vi "New plot.vi"() -> (0 "Boolean":bool)   [LabVIEW 2021]
uses:
  <vilib>/Utility/file.llb/Read Delimited Spreadsheet (string).vi
panel:
  out "filename":string
  out "VI Clone Name":string
  in  "file path (dialog if empty)":path
  out "XY Graph":cluster{dbl[], dbl[]}(graph)
  in  "stop":bool
  in  "Listbox":i32(listbox)
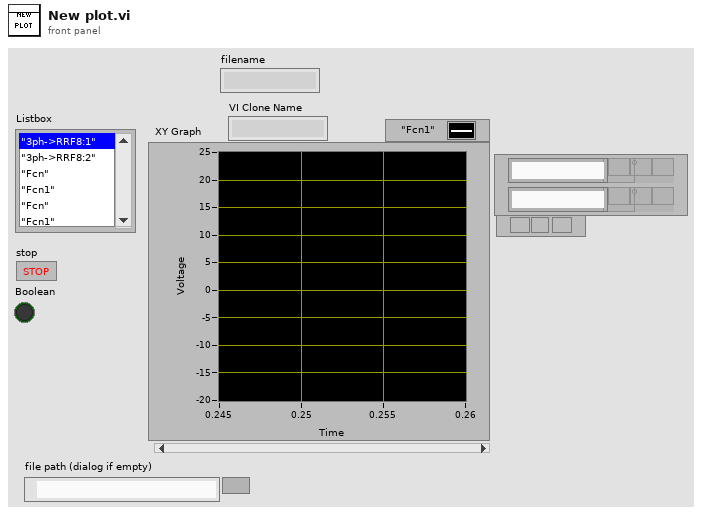
[diagram p1: front panel]
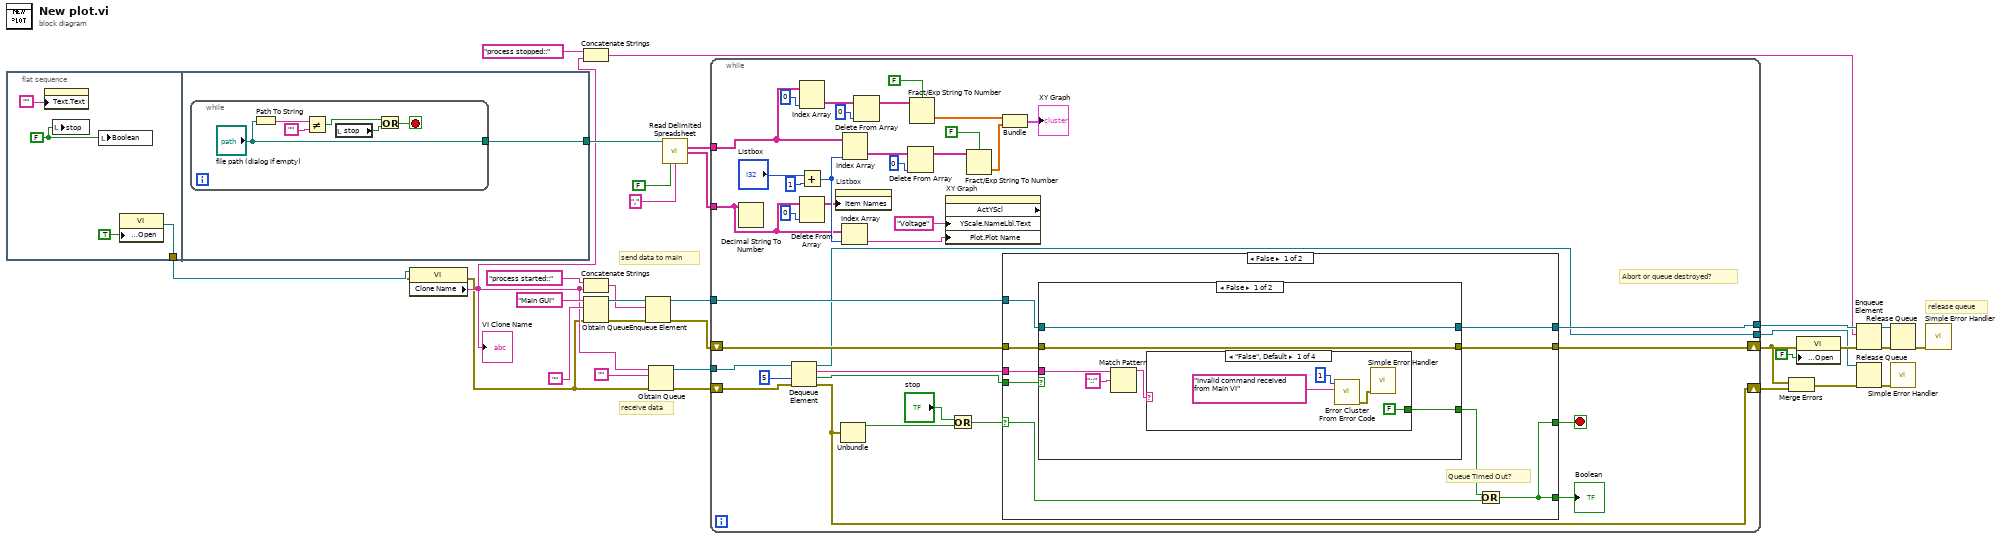
[diagram p0: block diagram]
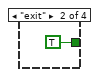
[diagram p2: hidden frame]
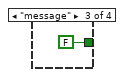
[diagram p3: hidden frame]
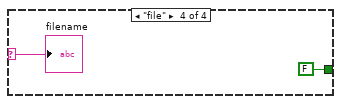
[diagram p4: hidden frame]
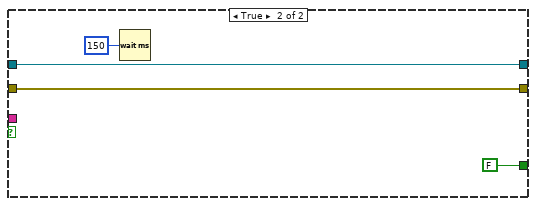
[diagram p5: hidden frame]
diagram:
  # "receive data"
  # "send data to main"
  # "release queue"
  n1 = flat-sequence {
    tunnel: [w35] -> w22
    tunnel: [w34] -> w21
    tunnel: [w39] -> w29
    frame #0 {
      w37 = FALSE ("stop")
      n2 = property on="file path (dialog if empty)" class="Path"("Text.Text"="") -> ()  [unwired: 2 in, 2 out]
      n3 = local write "stop"(w37) -> ()
      n4 = local write "Boolean"(w37) -> ()
      n5 = property class="VI"("Front Panel.Open"=TRUE ("Front Panel Window:Open")) -> (reference out=w35:refnum<vi>, error out=w34:errorcluster)  [unwired: 2 in]
    }
    frame #1 {
      n6 = while {
        tunnel: ["file path (dialog if empty)"] -> w39
        stop <- w40 stop-if-true
        n7 = Path To String(path="file path (dialog if empty)") -> (string=w43:string)
        n8 = Not Equal?(x=w43, y="") -> (x != y?=w41:bool)
        n9 = local read "stop"() -> (w42:bool)
        n10 = Or(x=w41, y=w42) -> (x .or. y?=w40:bool)
      }
    }
  }
  n11 = property class="VI"(reference=w22, error in=w21) -> (error out=w6:errorcluster, "Clone Name"=w9:string)  [unwired: 1 out]
  "VI Clone Name" <- w9
  n12 = Concatenate Strings("process stopped::" ("string"), w9) -> (w14:string)
  n13 = Concatenate Strings("process started::" ("name (unnamed)"), w9) -> (w23:string)
  n14 = Obtain Queue(name (unnamed)="Main GUI", element data type="", error in (no error)=w6) -> (queue out=w25:refnum<queue>, error out=w24:errorcluster)  [unwired: 2 in, 1 out]
  n15 = Enqueue Element(queue=w25, element=w23, error in (no error)=w24) -> (queue out=w20:refnum<queue>, error out=w19:errorcluster)  [unwired: 1 in, 1 out]
  n16 = Obtain Queue(name (unnamed)=w9, element data type="", error in (no error)=w6) -> (queue out=w8:refnum<queue>, error out=w7:errorcluster)  [unwired: 2 in, 1 out]
  n17 = call-poly <vilib>:"Read Delimited Spreadsheet.vi"("file path (dialog if empty)"=w29, "transpose? (F)"=FALSE, "delimiter (\\t)"="," ("delimiter (\\t)")) -> ("all rows"=w31:string[][], "first row"=w30:string[])  [unwired: 7 in, 4 out]
  n18 = while {
    tunnel: w31 -> [w74]
    tunnel: w30 -> [w64]
    tunnel: w20 -> [w59]
    tunnel: [w57] -> w18
    shift-right: [w56] -> w5
    shift-left: w19 -> [w58]
    tunnel: w8 -> [w55]
    tunnel: [w50] -> w3
    shift-right: [w49] -> w4
    shift-left: w7 -> [w48]
    stop <- w60 stop-if-true
    # "Abort or queue destroyed?"
    n19 = Decimal String To Number(string=w64) -> ()  [unwired: 2 in, 2 out]
    n20 = Dequeue Element(queue=w55, timeout in ms (-1)=5, error in (no error)=w48) -> (queue out=w50:refnum<queue>, element=w46:string, timed out?=w47:bool, error out=w49:errorcluster)
    n21 = Index Array(array=w74, index (col)=0 ("index (row)")) -> (element=w73:string[])  [unwired: 1 in]
    n22 = Add(x="Listbox", y=1) -> (x+y=w71:i32)
    n23 = Delete From Array(array=w64, index=0) -> (array with subset deleted=w63:string[])  [unwired: 1 in, 1 out]
    n24 = property on="Listbox" class="LstBox (strict)"("Item Names"=w63) -> ()  [unwired: 2 in, 2 out]
    n25 = Unbundle(w49) -> ("status"=w53:bool)  [unwired: 2 out]
    n26 = Index Array(array=w64, index=w71) -> (element=w69:string)
    n27 = Index Array(array=w74, index (col)=w71) -> (element=w78:string[])  [unwired: 1 in]
    n28 = Delete From Array(array=w73, index=0 ("index (col)")) -> (array with subset deleted=w76:string[])  [unwired: 1 in, 1 out]
    n29 = Delete From Array(array=w78, index=0) -> (array with subset deleted=w75:string[])  [unwired: 1 in, 1 out]
    n30 = Fract/Exp String To Number(use system decimal point (T)=FALSE, string=w76) -> (number=w70:dbl[])  [unwired: 2 in, 1 out]
    n31 = property on="XY Graph" class="XYGraph (strict)" props=["ActYScl", "YScale", "NameLbl", "Text", "Plot", "Plot Name"]("YScale.NameLbl.Text"="Voltage" ("Y Scale.Name Label.Text"), "Plot.Plot Name"=w69) -> ()  [unwired: 2 in, 3 out]
    n32 = Or(x="stop", y=w53) -> (x .or. y?=w52:bool)
    n33 = Fract/Exp String To Number(use system decimal point (T)=FALSE, string=w75) -> (number=w72:dbl[])  [unwired: 2 in, 1 out]
    n34 = Bundle(w70, w72) -> (→"XY Graph":cluster{dbl[], dbl[]})  [unwired: 1 in]
    n35 = case shown="False" w52 {
      selector: w52 -> [w88 w112]
      tunnel: [w87 w112] -> w61
      tunnel: [w87 w112] -> w60
      tunnel: w59 -> [w84 w111]
      tunnel: w58 -> [w86 w110]
      tunnel: [w83 w111] -> w57
      tunnel: [w85 w110] -> w56
      tunnel: w47 -> [w91 _]
      tunnel: w46 -> [w90 _]
      frame False {
        # "Queue Timed Out?"
        n36 = case shown="False" w91 {
          tunnel: w90 -> [w96 _]
          tunnel: [w94 FALSE] -> w89
          tunnel: w86 -> [w93 w109]
          tunnel: [w93 w109] -> w85
          tunnel: w84 -> [w92 w108]
          tunnel: [w92 w108] -> w83
          frame False {
            n37 = Match Pattern(string=w96, regular expression="::") -> (before substring=w97:string)  [unwired: 1 in, 3 out]
            n38 = case shown="\"False\", Default" w97 {
              selector: w97 -> [_ _ _ w105]
              tunnel: [FALSE TRUE FALSE FALSE] -> w94
              frame "False", Default {
                n39 = call <vilib>:"Error Cluster From Error Code.vi"("error message (\"\")"="Invalid command received from Main VI" ("error message (\"\")"), "error code (0)"=1) -> ("error out"=w99:errorcluster)  [unwired: 7 in]
                n40 = call <vilib>:"Simple Error Handler.vi"("error in (no error)"=w99) -> ()  [unwired: 4 in, 5 out]
              }
              frame "exit" {
              }
              frame "message" {
              }
              frame "file" {
                "filename" <- w105
              }
            }
          }
          frame True {
            n41 = Wait (ms)(milliseconds to wait=u32 150) -> ()  [unwired: 1 out]
          }
        }
        n42 = Or(x=w89, y=w88) -> (x .or. y?=w87:bool)
      }
      frame True {
      }
    }
    "Boolean" <- w61
  }
  n43 = Merge Errors(w5, w4) -> (w2:errorcluster)
  n44 = property class="VI"(error in=w5, "Front Panel.Open"=FALSE ("Front Panel Window:Open")) -> (error out=w12:errorcluster)  [unwired: 1 in, 1 out]
  n45 = Enqueue Element(queue=w18, element=w14, error in (no error)=w12) -> (queue out=w17:refnum<queue>, error out=w16:errorcluster)  [unwired: 1 in, 1 out]
  n46 = Release Queue(queue=w3, error in (no error)=w2) -> (error out=w1:errorcluster)  [unwired: 1 in, 2 out]
  n47 = Release Queue(queue=w17, error in (no error)=w16) -> (error out=w15:errorcluster)  [unwired: 1 in, 2 out]
  n48 = call <vilib>:"Simple Error Handler.vi"("error in (no error)"=w1) -> ()  [unwired: 4 in, 5 out]
  n49 = call <vilib>:"Simple Error Handler.vi"("error in (no error)"=w15) -> ()  [unwired: 4 in, 5 out]
